vi "Server.vi"() -> ()   [LabVIEW 2016]
uses:
  <vilib>/Utility/tcp.llb/UDP Multicast Write-Only Open.vi
panel:
  out "Users Ports":i32[](array[numeric])
  out "Users IPs":string[](array[string])
  in  "TransmissionMode":enum32{"MULTICAST", "UNICAST"}(radio)
  in  "MulticastAdress":string
  out "Index":i32
  out "AuthKeys":i32[](array[numeric])
  out "Array 3":string[][](array[string])
  out "Array":string[][](array[string])
  in  "Stop Button":bool
  out "Log":string
  in  "Add":bool
  out "Users List":string[][](table)
  # "User List"
  # "Multicast Address"
  # "Server Log"
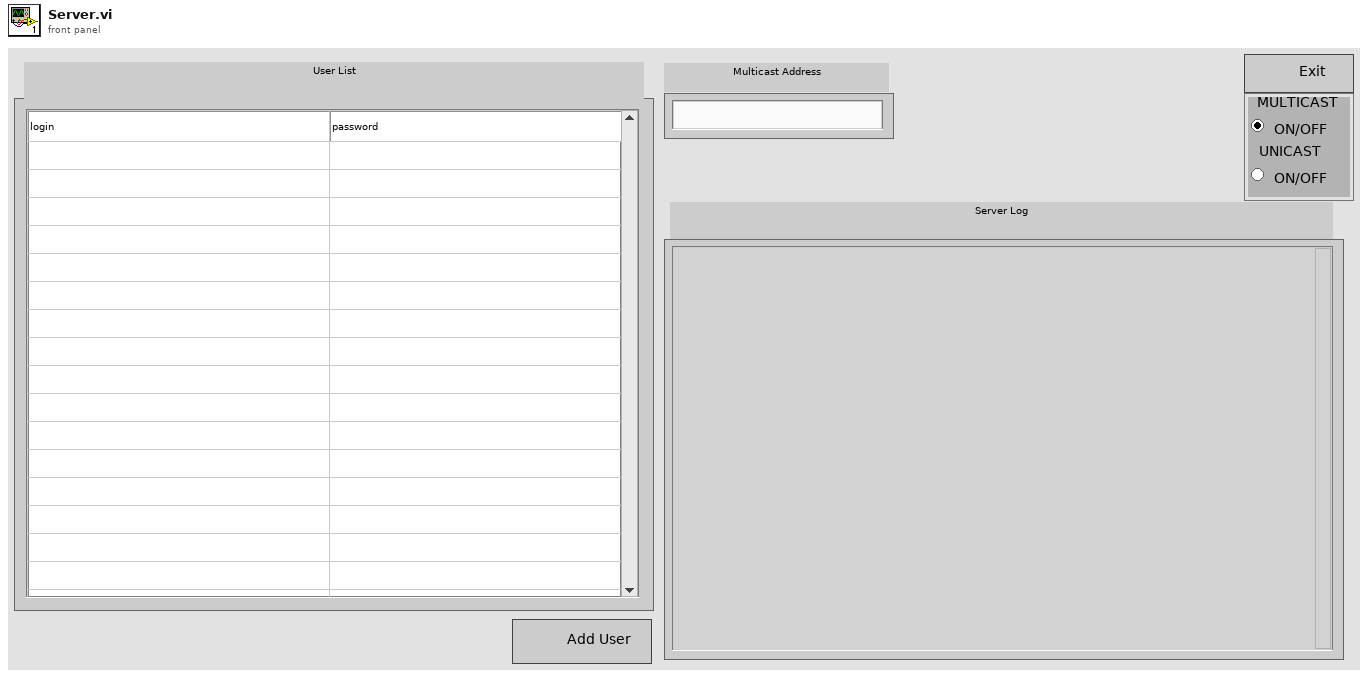
[diagram p1: front panel]
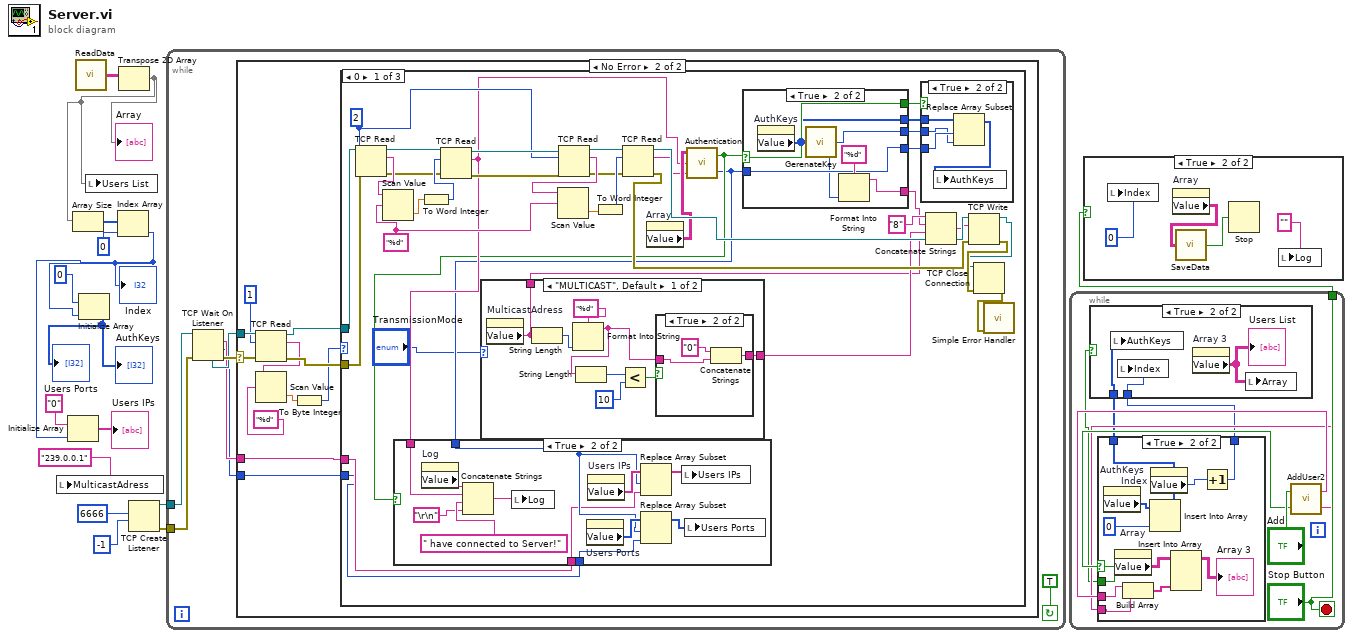
[diagram p0: block diagram]
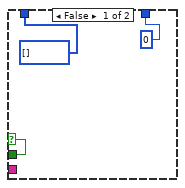
[diagram p4: hidden frame]
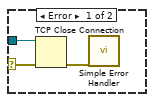
[diagram p5: hidden frame]
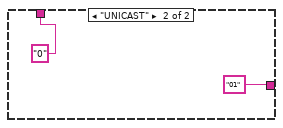
[diagram p7: hidden frame]
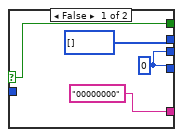
[diagram p10: hidden frame]
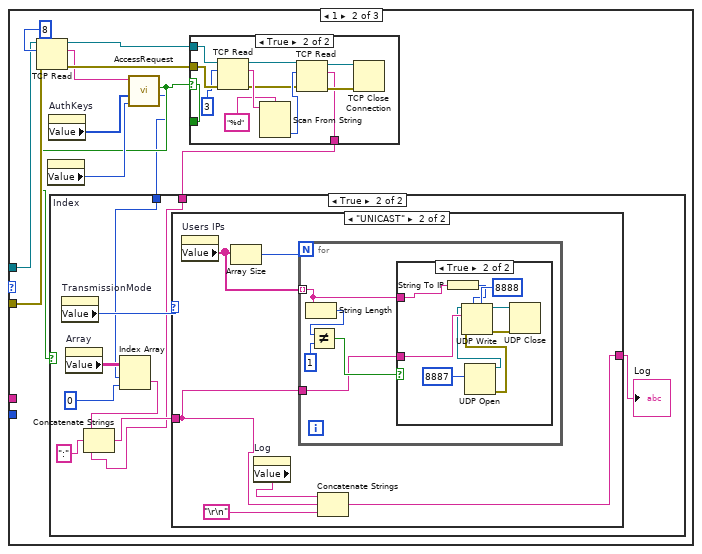
[diagram p11: hidden frame]
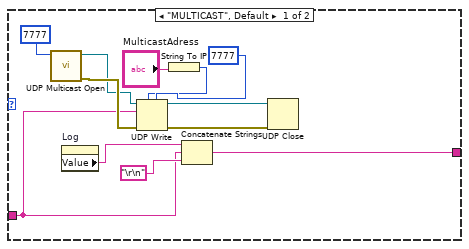
[diagram p13: hidden frame]
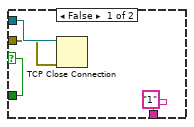
[diagram p15: hidden frame]
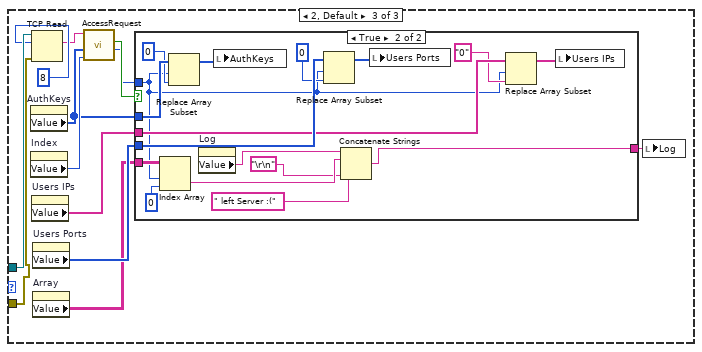
[diagram p16: hidden frame]
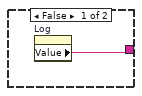
[diagram p17: hidden frame]
diagram:
  n1 = local write "MulticastAdress"("239.0.0.1") -> ()
  n2 = call "ReadData.vi"() -> ("Data"=w14:string[][])  [unwired: 1 in]
  n3 = Transpose 2D Array(2D array=w14) -> (transposed array=w9:string[][])
  "Array" <- w9
  n4 = Array Size(array=w9) -> (size(s)=w13:i32[])
  n5 = local write "Users List"(w9) -> ()
  n6 = Index Array(array=w13, index=0) -> (element=w7:i32)
  "Index" <- w7
  n7 = Initialize Array("0", w7) -> (→"Users IPs":string[])
  n8 = Initialize Array(0, w7) -> (→"AuthKeys" →"Users Ports":i32[])
  n9 = TCP Create Listener(9:-1, 10:6666) -> (0:w2:errorcluster, 3:w3:refnum<k5>)  [unwired: 3 in, 1 out]
  n10 = while {
    tunnel: w3 -> [w17]
    tunnel: w2 -> [w16]
    stop <- TRUE continue-if-true
    n11 = TCP Wait On Listener(8:w16, 11:w17) -> (0:w22:errorcluster, 1:w18:u16, 2:w19:string, 4:w21:refnum<k5>)  [unwired: 2 in, 1 out]
    n12 = case shown="No Error" w22 {
      selector: w22 -> [w25 w36]
      tunnel: w21 -> [w24 w35]
      tunnel: w19 -> [_ w27]
      tunnel: w18 -> [_ w26]
      frame Error {
        n13 = TCP Close Connection(connection ID=w24, error in (no error)=w25) -> (error out=w23:errorcluster)  [unwired: 1 in, 1 out]
        n14 = call <vilib>:"Simple Error Handler.vi"("error in (no error)"=w23) -> ()  [unwired: 4 in, 5 out]
      }
      frame No Error {
        n15 = TCP Read(connection ID=w35, bytes to read=1, error in (no error)=w36) -> (connection ID out=w32:refnum<k5>, data out=w30:string, error out=w31:errorcluster)  [unwired: 2 in]
        n16 = Scan Value(string=w30, format string="%d") -> (value=w29:dbl)  [unwired: 1 in, 1 out]
        n17 = To Byte Integer(number=w29) -> (8bit integer=w28:i8)
        n18 = case shown="0" w28 {
          tunnel: w32 -> [w58 w124 w194]
          tunnel: w31 -> [w57 w123 w185]
          tunnel: w27 -> [w44 _ _]
          tunnel: w26 -> [w43 _ _]
          frame 0 {
            w71 = "%d"
            w64 = 2
            n19 = TCP Read(connection ID=w58, bytes to read=w64, error in (no error)=w57) -> (connection ID out=w74:refnum<k5>, data out=w73:string, error out=w56:errorcluster)  [unwired: 2 in]
            n20 = Scan Value(string=w73, format string=w71) -> (value=w67:dbl)  [unwired: 1 in, 1 out]
            n21 = To Word Integer(number=w67) -> (16bit integer=w68:i16)
            n22 = TCP Read(connection ID=w74, bytes to read=w68, error in (no error)=w56) -> (connection ID out=w72:refnum<k5>, data out=w47:string, error out=w55:errorcluster)  [unwired: 2 in]
            n23 = case shown="\"MULTICAST\", Default" "TransmissionMode" {
              tunnel: [w76 "01"] -> w38
              tunnel: [w75 "0"] -> w37
              frame "MULTICAST", Default {
                n24 = property on="MulticastAdress" class="Str"() -> ("Value"=w75:string)  [unwired: 2 in, 2 out]
                n25 = String Length(string=w75) -> (length=w77:i32)
                n26 = Format Into String(format string="%d", w77) -> (resulting string=w82:string)  [unwired: 2 in, 1 out]
                n27 = String Length(string=w82) -> (length=w79:i32)
                n28 = Less?(x=w79, y=10) -> (x < y?=w81:bool)
                n29 = case shown="True" w81 {
                  tunnel: w82 -> [w83 w85]
                  tunnel: [w83 w84] -> w76
                  frame False {
                  }
                  frame True {
                    n30 = Concatenate Strings("0", w85) -> (w84:string)
                  }
                }
              }
              frame "UNICAST" {
              }
            }
            n31 = TCP Read(connection ID=w72, bytes to read=w64, error in (no error)=w55) -> (connection ID out=w69:refnum<k5>, data out=w70:string, error out=w54:errorcluster)  [unwired: 2 in]
            n32 = Scan Value(string=w70, format string=w71) -> (value=w66:dbl)  [unwired: 1 in, 1 out]
            n33 = To Word Integer(number=w66) -> (16bit integer=w65:i16)
            n34 = TCP Read(connection ID=w69, bytes to read=w65, error in (no error)=w54) -> (connection ID out=w60:refnum<k5>, data out=w51:string, error out=w53:errorcluster)  [unwired: 2 in]
            n35 = property on="Array" class="Arr (strict)"() -> ("Value"=w52:string[][])  [unwired: 2 in, 2 out]
            n36 = call "Authentication.vi"("password"=w51, "login"=w47, "Server Data"=w52) -> ("Index"=w45:i32, "IsValid?"=w46:bool)
            n37 = case shown="True" w46 {
              tunnel: w47 -> [_ w100]
              tunnel: w45 -> [_ w93]
              tunnel: w44 -> [_ w92]
              tunnel: w43 -> [_ w91]
              frame False {
              }
              frame True {
                n38 = property on="Log" class="Str"() -> ("Value"=w97:string)  [unwired: 2 in, 2 out]
                n39 = Concatenate Strings(w97, w100, " have connected to Server!", "\r\n") -> (w96:string)
                n40 = local write "Log"(w96) -> ()
                n41 = property on="Users Ports" class="Arr (strict)"() -> ("Value"=w94:i32[])  [unwired: 2 in, 2 out]
                n42 = property on="Users IPs" class="Arr (strict)"() -> ("Value"=w95:string[])  [unwired: 2 in, 2 out]
                n43 = Replace Array Subset(array=w95, new element=w92, index=w93) -> (w90:string[])
                n44 = Replace Array Subset(array=w94, new element=w91, index=w93) -> (w89:i32[])
                n45 = local write "Users IPs"(w90) -> ()
                n46 = local write "Users Ports"(w89) -> ()
              }
            }
            n47 = case shown="True" w46 {
              selector: w46 -> [w108 w114]
              tunnel: [w108 w114] -> w63
              tunnel: [i32[] [] w111] -> w62
              tunnel: w45 -> [_ w112]
              tunnel: [w106 w112] -> w50
              tunnel: [w106 w110] -> w49
              tunnel: ["00000000" w109] -> w48
              frame False {
                w106 = 0
              }
              frame True {
                n48 = property on="AuthKeys" class="Arr (strict)"() -> ("Value"=w111:i32[])  [unwired: 2 in, 2 out]
                n49 = call "GerenateKey.vi"("Array"=w111) -> ("Numeric"=w110:i32)
                n50 = Format Into String(format string="%d", w110) -> (resulting string=w109:string)  [unwired: 2 in, 1 out]
              }
            }
            n51 = case shown="True" w63 {
              tunnel: w62 -> [_ w102]
              tunnel: w50 -> [_ w104]
              tunnel: w49 -> [_ w103]
              frame False {
              }
              frame True {
                n52 = Replace Array Subset(array=w102, new element=w103, index=w104) -> (w101:i32[])
                n53 = local write "AuthKeys"(w101) -> ()
              }
            }
            n54 = Concatenate Strings("8", w48, w38, w37) -> (w59:string)
            n55 = TCP Write(connection ID=w60, data in=w59, error in (no error)=w53) -> (connection ID out=w39:refnum<k5>, error out=w40:errorcluster)  [unwired: 1 in, 1 out]
            n56 = TCP Close Connection(connection ID=w39, error in (no error)=w40) -> (error out=w41:errorcluster)  [unwired: 1 in, 1 out]
            n57 = call <vilib>:"Simple Error Handler.vi"("error in (no error)"=w41) -> ()  [unwired: 4 in, 5 out]
          }
          frame 1 {
            n58 = TCP Read(connection ID=w124, bytes to read=8, error in (no error)=w123) -> (connection ID out=w120:refnum<k5>, data out=w118:string, error out=w119:errorcluster)  [unwired: 2 in]
            n59 = property on="Index" class="DigNum (strict)"() -> ("Value"=w121:i32)  [unwired: 2 in, 2 out]
            n60 = property on="AuthKeys" class="Arr (strict)"() -> ("Value"=w122:i32[])  [unwired: 2 in, 2 out]
            n61 = call "AccessRequest.vi"("Index"=w121, "KeyList"=w122, "InputKey"=w118) -> ("UserID"=w116:i32, "IsAccess?"=w117:bool)  [unwired: 7 in]
            n62 = case shown="True" w117 {
              selector: w117 -> [w168 w172]
              tunnel: w120 -> [w170 w182]
              tunnel: w119 -> [w169 w181]
              tunnel: [w168 w172] -> _
              tunnel: ["1" w171] -> w115
              frame False {
                n63 = TCP Close Connection(connection ID=w170, error in (no error)=w169) -> ()  [unwired: 1 in, 2 out]
              }
              frame True {
                n64 = TCP Read(connection ID=w182, bytes to read=3, error in (no error)=w181) -> (connection ID out=w176:refnum<k5>, data out=w179:string, error out=w175:errorcluster)  [unwired: 2 in]
                n65 = Scan From String(format string="%d", input string=w179) -> (output 1=w177:i32)  [unwired: 3 in, 3 out]
                n66 = TCP Read(connection ID=w176, bytes to read=w177, error in (no error)=w175) -> (connection ID out=w173:refnum<k5>, data out=w171:string, error out=w174:errorcluster)  [unwired: 2 in]
                n67 = TCP Close Connection(connection ID=w173, error in (no error)=w174) -> ()  [unwired: 1 in, 2 out]
              }
            }
            n68 = case shown="True" w117 {
              tunnel: w116 -> [_ w129]
              tunnel: w115 -> [_ w127]
              frame False {
              }
              frame True {
                n69 = property on="TransmissionMode" class="RadioBtnsControl (strict)"() -> ("Value"=w134:enum32{"MULTICAST", "UNICAST"})  [unwired: 2 in, 2 out]
                n70 = property on="Array" class="Arr (strict)"() -> ("Value"=w132:string[][])  [unwired: 2 in, 2 out]
                n71 = Index Array(array=w132, index (row)=w129, index (col)=0) -> (element=w128:string)
                n72 = Concatenate Strings(w128, ":", w127) -> (w130:string)
                n73 = case shown="\"UNICAST\"" w134 {
                  tunnel: w130 -> [w137 w149]
                  tunnel: [w136 w148] -> w126
                  frame "MULTICAST", Default {
                    n74 = call-poly <vilib>:"UDP Multicast Open.vi"("port"=7777) -> ("error out"=w138:errorcluster, "connection ID"=w135:refnum<k16>)  [unwired: 9 in]
                    n75 = property on="Log" class="Str"() -> ("Value"=w145:string)  [unwired: 2 in, 2 out]
                    n76 = String To IP(1:"MulticastAdress") -> (0:w140:u32)
                    n77 = UDP Write(address=w140, port or service name=7777, connection ID=w135, data in=w137, 8:w138) -> (error out=w143:errorcluster, 3:w142:refnum<k16>)  [unwired: 1 in]
                    n78 = Concatenate Strings(w145, w137, "\r\n") -> (w136:string)
                    n79 = UDP Close(connection ID=w142, 8:w143) -> ()  [unwired: 2 out]
                  }
                  frame "UNICAST" {
                    n80 = property on="Users IPs" class="Arr (strict)"() -> ("Value"=w152:string[])  [unwired: 2 in, 2 out]
                    n81 = Array Size(array=w152) -> (size(s)=w147:i32)
                    n82 = property on="Log" class="Str"() -> ("Value"=w151:string)  [unwired: 2 in, 2 out]
                    n83 = for {
                      N: w147 -> [_]
                      tunnel: w152 -> [w155] mode=indexing
                      tunnel: w149 -> [w154]
                      n84 = String Length(string=w155) -> (length=w153:i32)
                      n85 = Not Equal?(x=w153, y=1) -> (x != y?=w156:bool)
                      n86 = case shown="True" w156 {
                        tunnel: w155 -> [_ w165]
                        tunnel: w154 -> [_ w166]
                        frame False {
                        }
                        frame True {
                          n87 = String To IP(1:w165) -> (0:w161:u32)
                          n88 = UDP Open(11:8887) -> (port=w159:refnum<k16>, 0:w158:errorcluster)  [unwired: 4 in, 1 out]
                          n89 = UDP Write(address=w161, port or service name=8888, connection ID=w159, data in=w166, 8:w158) -> (error out=w164:errorcluster, 3:w163:refnum<k16>)  [unwired: 1 in]
                          n90 = UDP Close(connection ID=w163, 8:w164) -> ()  [unwired: 2 out]
                        }
                      }
                    }
                    n91 = Concatenate Strings(w151, w149, "\r\n") -> (w148:string)
                  }
                }
                "Log" <- w126
              }
            }
          }
          frame 2, Default {
            n92 = property on="AuthKeys" class="Arr (strict)"() -> ("Value"=w188:i32[])  [unwired: 2 in, 2 out]
            n93 = property on="Index" class="DigNum (strict)"() -> ("Value"=w191:i32)  [unwired: 2 in, 2 out]
            n94 = TCP Read(connection ID=w194, bytes to read=8, error in (no error)=w185) -> (data out=w192:string)  [unwired: 2 in, 2 out]
            n95 = property on="Users IPs" class="Arr (strict)"() -> ("Value"=w187:string[])  [unwired: 2 in, 2 out]
            n96 = property on="Users Ports" class="Arr (strict)"() -> ("Value"=w186:i32[])  [unwired: 2 in, 2 out]
            n97 = property on="Array" class="Arr (strict)"() -> ("Value"=w184:string[][])  [unwired: 2 in, 2 out]
            n98 = call "AccessRequest.vi"("Index"=w191, "KeyList"=w188, "InputKey"=w192) -> ("UserID"=w189:i32, "IsAccess?"=w190:bool)  [unwired: 7 in]
            n99 = case shown="True" w190 {
              tunnel: w189 -> [_ w202]
              tunnel: w188 -> [_ w212]
              tunnel: w187 -> [_ w206]
              tunnel: w186 -> [_ w209]
              tunnel: w184 -> [_ w203]
              tunnel: [w195 w197] -> w183
              frame False {
                n100 = property on="Log" class="Str"() -> ("Value"=w195:string)  [unwired: 2 in, 2 out]
              }
              frame True {
                n101 = Index Array(array=w203, index (row)=w202, index (col)=0) -> (element=w199:string)
                n102 = Replace Array Subset(array=w212, new element=0, index=w202) -> (w210:i32[])
                n103 = property on="Log" class="Str"() -> ("Value"=w200:string)  [unwired: 2 in, 2 out]
                n104 = local write "AuthKeys"(w210) -> ()
                n105 = Replace Array Subset(array=w209, new element=0, index=w202) -> (w207:i32[])
                n106 = Concatenate Strings(w200, w199, " left Server :(", "\r\n") -> (w197:string)
                n107 = local write "Users Ports"(w207) -> ()
                n108 = Replace Array Subset(array=w206, new element="0", index=w202) -> (w204:string[])
                n109 = local write "Users IPs"(w204) -> ()
              }
            }
            n110 = local write "Log"(w183) -> ()
          }
        }
      }
    }
  }
  n111 = while {
    tunnel: ["Stop Button"] -> w10
    stop <- "Stop Button" stop-if-true
    n112 = call "AddUser2.vi"("Add?"="Add") -> ("password"=w216:string, "login"=w217:string, "Success?"=w218:bool)
    n113 = case shown="True" w218 {
      selector: w218 -> [w226 w233]
      tunnel: w216 -> [_ w237]
      tunnel: [w226 w233] -> w215
      tunnel: w217 -> [_ w232]
      tunnel: [0 w228] -> w214
      tunnel: [i32[] [] w227] -> w213
      frame False {
      }
      frame True {
        n114 = property on="AuthKeys" class="Arr (strict)"() -> ("Value"=w230:i32[])  [unwired: 2 in, 2 out]
        n115 = property on="Array" class="Arr (strict)"() -> ("Value"=w236:string[][])  [unwired: 2 in, 2 out]
        n116 = Build Array(w232, w237) -> (w235:string[])
        n117 = Insert Into Array(array=w230, new element=0) -> (w227:i32[])  [unwired: 1 in]
        n118 = property on="Index" class="DigNum (strict)"() -> ("Value"=w229:i32)  [unwired: 2 in, 2 out]
        n119 = Insert Into Array(array=w236, new element=w235) -> (→"Array 3":string[][])  [unwired: 2 in]
        n120 = Increment(x=w229) -> (x+1=w228:i32)
      }
    }
    n121 = case shown="True" w215 {
      tunnel: w214 -> [_ w221]
      tunnel: w213 -> [_ w222]
      frame False {
      }
      frame True {
        n122 = local write "AuthKeys"(w222) -> ()
        n123 = local write "Index"(w221) -> ()
        n124 = property on="Array 3" class="Arr (strict)"() -> ("Value"=w223:string[][])  [unwired: 2 in, 2 out]
        "Users List" <- w223
        n125 = local write "Array"(w223) -> ()
      }
    }
  }
  n126 = case shown="True" w10 {
    frame False {
    }
    frame True {
      n127 = local write "Index"(0) -> ()
      n128 = property on="Array" class="Arr (strict)"() -> ("Value"=w241:string[][])  [unwired: 2 in, 2 out]
      n129 = call "SaveData.vi"("Input 2D Array"=w241) -> ("Success?"=w240:bool)
      n130 = Stop(stop? (T)=w240) -> ()
      n131 = local write "Log"("") -> ()
    }
  }
